vi "Detect Chassis.vi"(8 "error in":errorcluster, 11 "Controller in":refnum<class "Controller.lvclass">) -> (0 "error out":errorcluster, 3 "Controller out":refnum<class "Controller.lvclass">)   [LabVIEW 2015, in "SMI.lvlib" / "Controller.lvclass"]
uses:
  Controller.lvclass
  SysCfg Device/SysCfg Device.lvclass/SysCfg Device.ctl
  Controller.lvclass/Controller.ctl
  SysCfg Device/Accessor Methods/Read SysCfg Session.vi
  SysCfg Device/Accessor Methods/Write SysCfg Session.vi
  Chassis/Chassis.lvclass
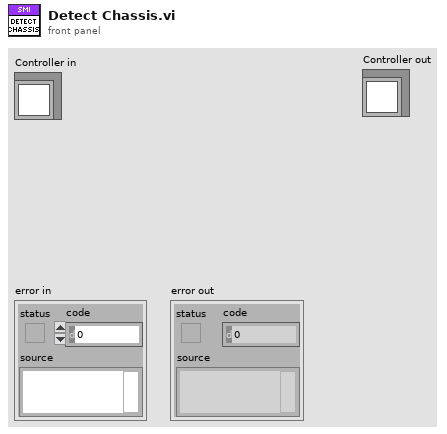
[diagram p1: front panel]
types:
  T1 = typedef "SMI.lvlib/Chassis.lvclass/ChassisInformation.ctl" = cluster{"Resource Name":string, "Vendor Name":string, "Product Name":string, "Product ID":u16, "Serial Number":string, "Number of Slots":i32}
  T2 = cluster{"Local Chassis":T1[], "Remote Chassis":T1[]}
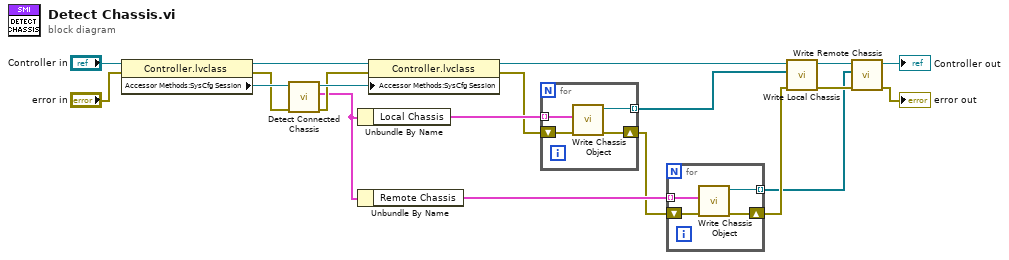
[diagram p0: block diagram]
diagram:
  n1 = property class="Controller.lvclass"(reference="Controller in", error in="error in") -> (reference out=w17:refnum<class "Controller.lvclass">, error out=w19:errorcluster, "Accessor Methods:SysCfg Session"=w20:refnum<k21>)
  n2 = call "Detect Connected Chassis.vi"("error in"=w19, "SysCfg Session in"=w20) -> ("error out"=w15:errorcluster, "Chassis"=w9:T2, "SysCfg Session out"=w16:refnum<k21>)  [unwired: 7 in]
  n3 = Unbundle By Name(w9) -> ("Local Chassis"=w7:T1[])
  n4 = Unbundle By Name(w9) -> ("Remote Chassis"=w8:T1[])
  n5 = property class="Controller.lvclass"(reference=w17, error in=w15, "Accessor Methods:SysCfg Session"=w16) -> (reference out=w1:refnum<class "Controller.lvclass">, error out=w6:errorcluster)
  n6 = for {
    tunnel: w7 -> [w24] mode=indexing
    shift-right: [w22] -> w5
    shift-left: w6 -> [w23]
    tunnel: [w21] -> w4 mode=indexing
    n7 = call "Write Chassis Object.vi"("error in"=w23, "Chassis Information"=w24) -> ("error out"=w22:errorcluster, "Chassis out"=w21:refnum<class "Chassis.lvclass">)  [unwired: 8 in]
  }
  n8 = for {
    tunnel: w8 -> [w28] mode=indexing
    shift-right: [w26] -> w10
    shift-left: w5 -> [w27]
    tunnel: [w25] -> w3 mode=indexing
    n9 = call "Write Chassis Object.vi"("error in"=w27, "Chassis Information"=w28) -> ("error out"=w26:errorcluster, "Chassis out"=w25:refnum<class "Chassis.lvclass">)  [unwired: 8 in]
  }
  n10 = call "Write Local Chassis.vi"("error in (no error)"=w10, "Local Chassis"=w4, "Controller in"=w1) -> ("error out"=w11:errorcluster, "Controller out"=w14:refnum<class "Controller.lvclass">)  [unwired: 7 in]
  n11 = call "Write Remote Chassis.vi"("error in (no error)"=w11, "Remote Chassis"=w3, "Controller in"=w14) -> ("error out"=→"error out":errorcluster, "Controller out"=→"Controller out":refnum<class "Controller.lvclass">)  [unwired: 7 in]
